vi "Untitled 4.vi"() -> ()   [LabVIEW 2016]
panel:
  in  "Mask":dbl[][](graph)=array180x1000[180000 elements]
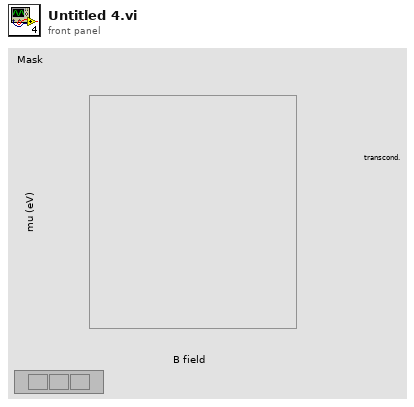
[diagram p1: front panel]
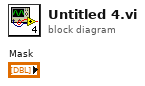
[diagram p0: block diagram]
diagram:
